vi "PID (Compatibility).vi"(4 "iteration":i32, 6 "options":T1={"sp low"=0.0, "sp high"=100.0, "out low"=-100.0, "out high"=100.0, "hold (F)"=FALSE, "auto (T)"=TRUE, "pro. band (F)"=FALSE, "reverse acting (T)"=TRUE, "beta"=1.0, "linearity"=1.0, "dt (s)"=-1.0} {"dt (s)" format="%.2f"; "linearity" min=0.0 max=1.0 format="%.2f"; "sp low" format="%.2f"; "sp high" format="%.2f"; "out low" format="%.2f"; "out high" format="%.2f"; "beta" min=0.0 max=1.0 format="%.2f"}, 8 "manual control":dbl format="%.2f", 9 "PID parameters":cluster{"Kp":dbl, "Ti":dbl, "Td":dbl} {"Td" format="%.2f"; "Ti" format="%.2f"; "Kp" format="%.2f"}, 10 "process variable":dbl format="%.2f", 11 "setpoint":dbl format="%.2f") -> (3 "output":dbl format="%.2f")   [LabVIEW 2020, in "NI_PID__prctrl compat.lvlib"]
doc: "Implements a PID controller using a PID algorithm for simple PID applications or high speed control applications that require an efficient algorithm. The PID algorithm features control output range limiting with integrator anti-windup and bumpless controller output for PID gain changes. Use the DBL instance of this VI to implement a single control loop. Use the DBL Array instance to implement parallel multi-loop control."
uses:
  NI_PID__prctrl compat.lvlib
panel:
  # "PID Controller"
  # "SP & PV range:"
  # "Output range:"
  # "-1: default,using system clock"
  # "Proportional gain or band (Kc)"
  # "Integral (reset) time (Ti, min)"
  # "Derivative (rate) time (Td, min)"
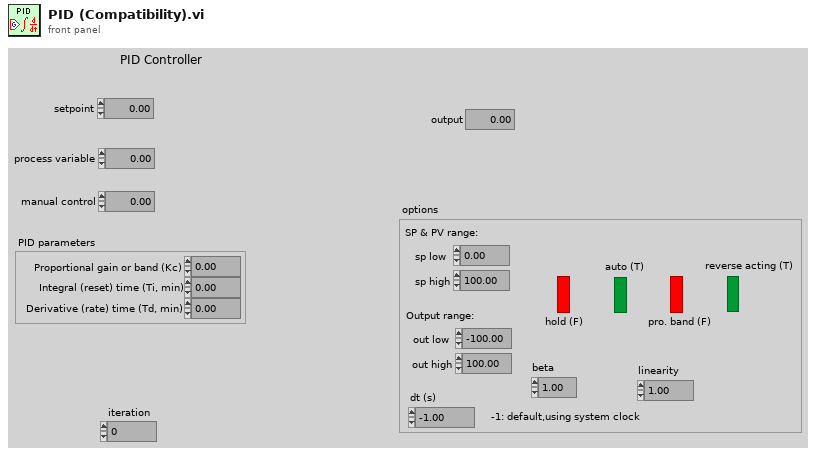
[diagram p1: front panel]
types:
  T1 = cluster{"sp low":dbl, "sp high":dbl, "out low":dbl, "out high":dbl, "hold (F)":bool, "auto (T)":bool, "pro. band (F)":bool, "reverse acting (T)":bool, "beta":dbl, "linearity":dbl, "dt (s)":dbl}
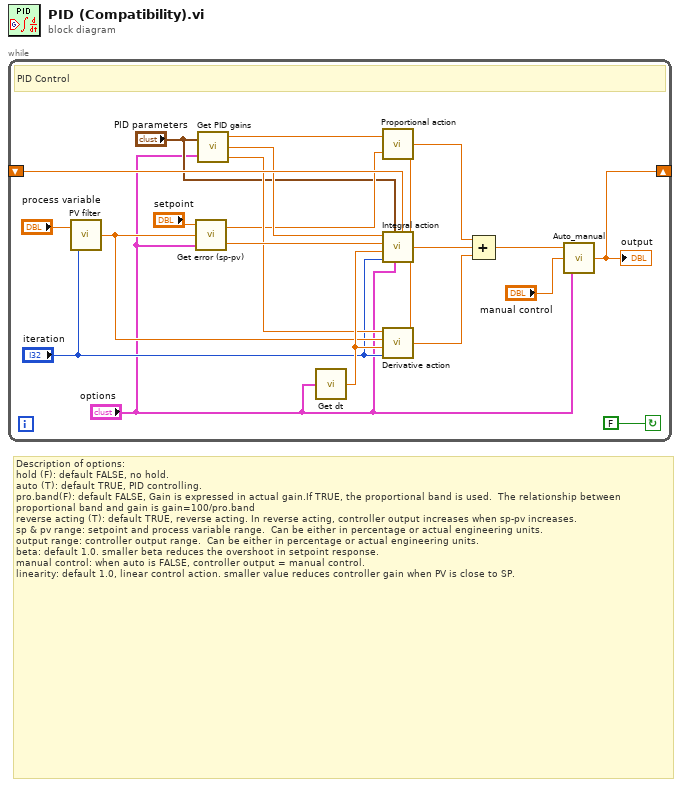
[diagram p0: block diagram]
diagram:
  # "Description of options:\nhold (F): default FALSE, no hold.\nauto (T): default TRUE, PID controlling.\npro.band(F): default FALSE, Gain is expressed in actual gain.If TRUE, the proportional band is used.  The relationship between proportional band and gain is gain=100/pro.band \nreverse acting (T): default TRUE, reverse acting. In reverse acting, controller output increases when sp-pv increases. \nsp & pv range: setpoint and process variable range.  Can be either in percentage or actual engineering units. \noutput range: controller output range.  Can be either in percentage or actual engineering units.\nbeta: default 1.0. smaller beta reduces the overshoot in setpoint response.\nmanual control: when auto is FALSE, controller output = manual control.\nlinearity: default 1.0, linear control action. smaller value reduces controller gain when PV is close to SP."
  n1 = while {
    shift-left: _ -> [w20]
    shift-right: [w6] -> _
    stop <- FALSE continue-if-true
    # "PID Control"
    n2 = call "PV filter.vi"("iteration"="iteration", "process variable"="process variable") -> ("filtered pv"=w15:dbl)
    n3 = call "Get error (sp-pv).vi"("options"="options", "process variable"=w15, "setpoint"="setpoint") -> ("error"=w14:dbl, "error (with beta)"=w10:dbl)
    n4 = call "Get PID gains.vi"("PID parameters"="PID parameters", "options"="options") -> ("Kc"=w11:dbl, "Ki"=w12:dbl, "Kd"=w13:dbl)
    n5 = call "Get dt.vi"("options"="options") -> ("dt (min.)"=w16:dbl)
    n6 = call "Proportional action.vi"("error"=w10, "Kc"=w11) -> ("proportional action"=w19:dbl)
    n7 = call "Derivative action.vi"("iteration"="iteration", "dt"=w16, "process variable"=w15, "Kd"=w13) -> ("derivative action"=w18:dbl)
    n8 = call "Integral action.vi"("derivative action"=w18, "proportional action"=w19, "prev. control output"=w20, "options"="options", "PID parameters"="PID parameters", "iteration"="iteration", "dt"=w16, "error"=w14, "Ki"=w12) -> ("integral action"=w17:dbl)  [unwired: 2 out]
    n9 = Compound Arithmetic op=ADD(w19, w17, w18) -> (w8:dbl)
    n10 = call "Auto_manual.vi"("options"="options", "manual control"="manual control", "auto control"=w8) -> ("output"=w6:dbl)
    "output" <- w6
  }
